vi "Channel 0 Individual Tube check (Reperpouse for Brute Force).vi"(0 "VISA Refnum in":refnum<visa-resource-name>, 1 "Test?":bool, 2 "Channel # in":i32, 3 "BoardHandle in":T1, 5 "Array":dbl[](array[numeric]), 7 "error in (no error)":errorcluster, 8 "Barcodes in":string[](array[string]), 11 "Tube #":i32) -> (12 "Next Measurment":string, 14 "Recorded Current\nfor Previous Tube":dbl format="%#_13g", 16 "Actual Voltage Level (V) 2":dbl format="%#_13g")   [LabVIEW 2020]
uses:
  <instrlib>/CAEN PSM/CAEN PSM.lvlib
panel:
  out "Failed Tubes":string[](array[string])
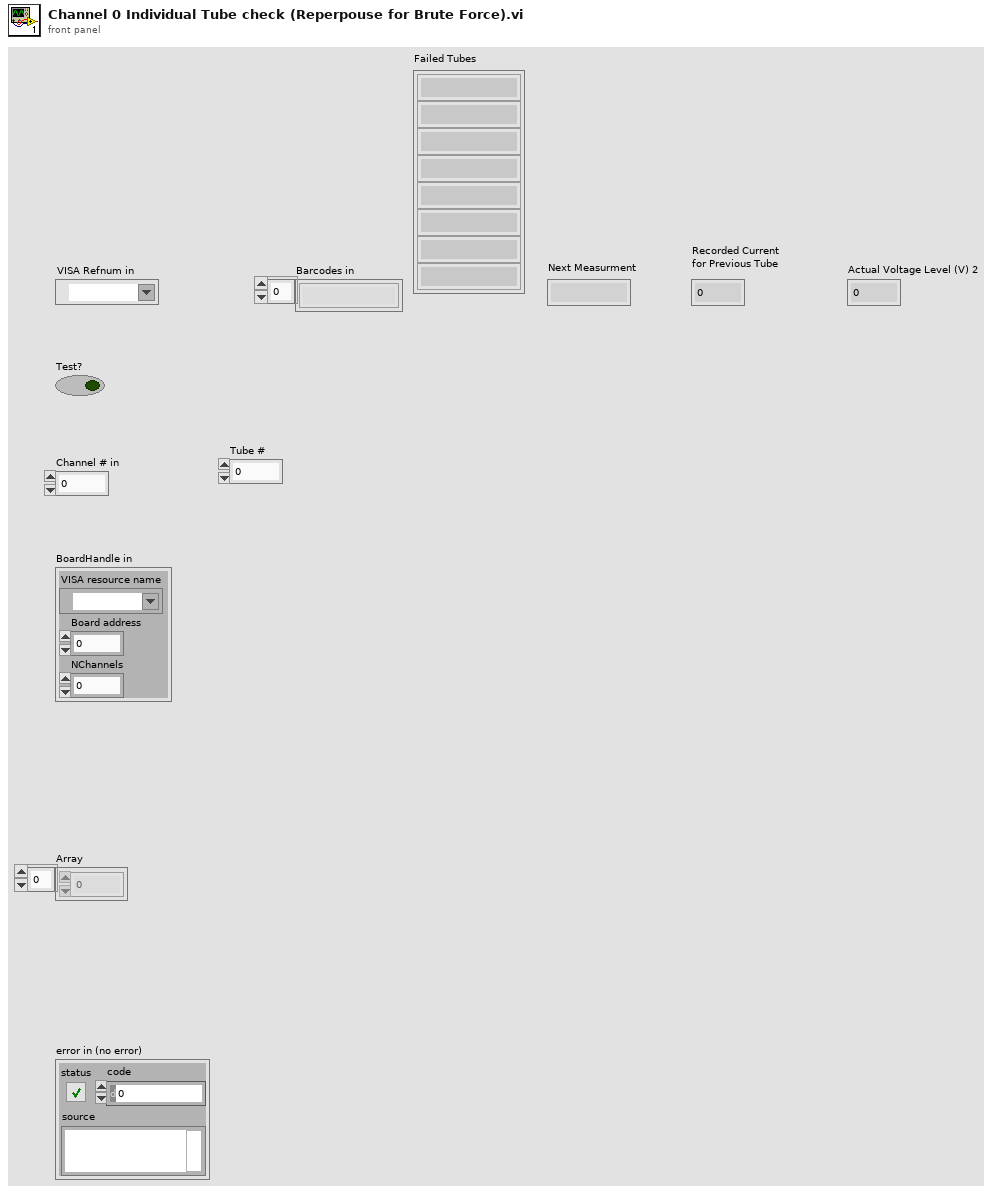
[diagram p1: front panel]
types:
  T1 = cluster{"VISA resource name":refnum<visa-resource-name>, "Board address":u8, "NChannels":u8}
  T2 = cluster{"ON":bool, "RUP":bool, "RDW":bool, "OVC":bool, "OVV":bool, "UNV":bool, "MAXV":bool, "TRIP":bool, "OVP":bool, "OVT":bool, "DIS":bool, "KILL":bool, "ILK":bool, "NOCAL":bool}[]
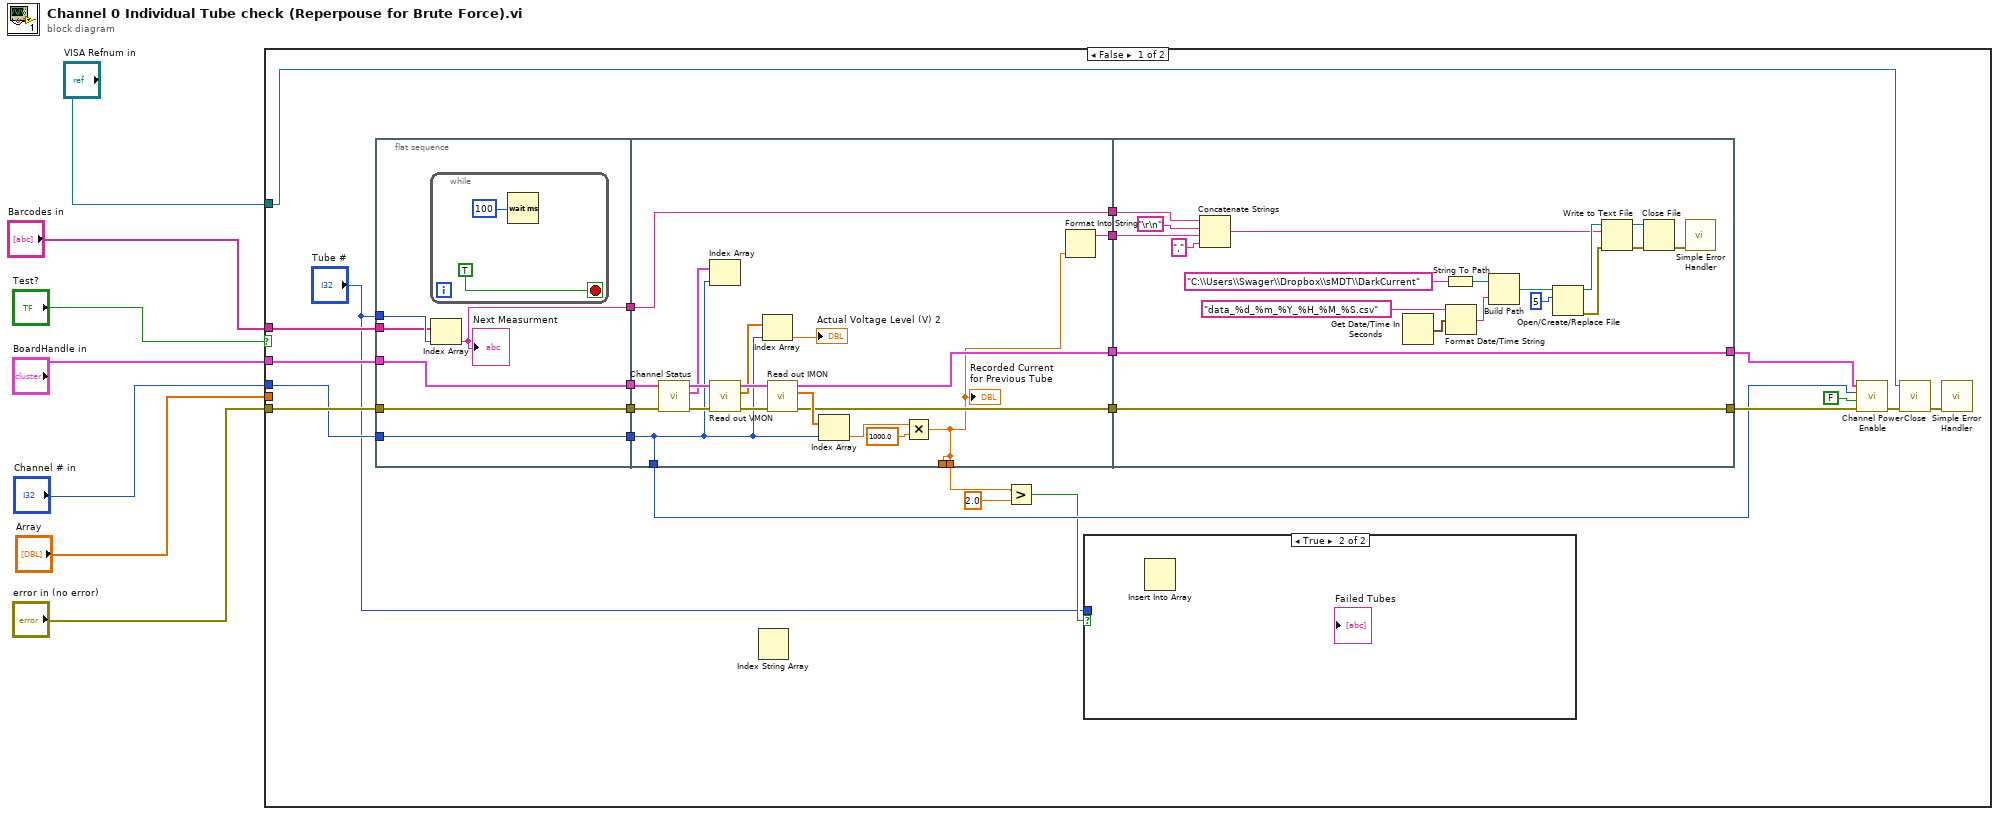
[diagram p0: block diagram]
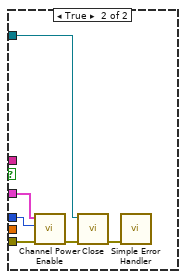
[diagram p3: hidden frame]
diagram:
  n1 = case shown="False" "Test?" {
    tunnel: "BoardHandle in" -> [w29 w78]
    tunnel: "error in (no error)" -> [w30 w77]
    tunnel: "Channel # in" -> [w28 w76]
    tunnel: "VISA Refnum in" -> [w24 w79]
    tunnel: "Array" -> [_ _]
    tunnel: "Barcodes in" -> [w20 _]
    frame False {
      n2 = flat-sequence {
        tunnel: "Tube #" -> [w36]
        tunnel: [w35] -> w19
        tunnel: w28 -> [w34]
        tunnel: [w34] -> w18
        tunnel: [w33] -> w17
        tunnel: w29 -> [w33]
        tunnel: [w32] -> w16
        tunnel: w30 -> [w32]
        tunnel: w20 -> [w31]
        tunnel: w19 -> [w46]
        tunnel: [w46] -> w15
        tunnel: w18 -> [w41]
        tunnel: w17 -> [w44]
        tunnel: w16 -> [w45]
        tunnel: [w43] -> w14
        tunnel: [w42] -> w13
        tunnel: [w41] -> w21
        tunnel: [w40] -> w12
        tunnel: [w39] -> w11
        tunnel: [w39] -> _
        tunnel: w15 -> [w61]
        tunnel: w14 -> [w59]
        tunnel: w13 -> [w58]
        tunnel: [w59] -> w23
        tunnel: [w58] -> w22
        tunnel: w12 -> [w57]
        frame #0 {
          n3 = while {
            stop <- TRUE ("Measure Next Tube") stop-if-true
            n4 = Wait (ms)(milliseconds to wait=100) -> ()  [unwired: 1 out]
          }
          n5 = Index Array(array=w31, index=w36) -> (element=w35:string)
          "Next Measurment" <- w35
        }
        frame #1 {
          n6 = call <instrlib>:"Channel Status.vi"("error in (no error)"=w45, "BoardHandle"=w44) -> ("error out"=w49:errorcluster, "Channel Status Array"=w48:T2, "BoardHandle out"=w50:T1)  [unwired: 7 in]
          n7 = Index Array(array=w48, index=w41) -> ()  [unwired: 1 out]
          n8 = call <instrlib>:"Read out VMON.vi"("error in (no error)"=w49, "BoardHandle"=w50) -> ("error out"=w53:errorcluster, "VMon values (V)"=w51:dbl[], "BoardHandle out"=w52:T1)  [unwired: 7 in]
          n9 = Index Array(array=w51, index=w41) -> (element=→"Actual Voltage Level (V) 2":dbl)
          n10 = call <instrlib>:"Read out IMON.vi"("error in (no error)"=w53, "BoardHandle"=w52) -> ("error out"=w42:errorcluster, "IMon values (uA)"=w56:dbl[], "BoardHandle out"=w43:T1)  [unwired: 6 in, 1 out]
          n11 = Index Array(array=w56, index=w41) -> (element=w54:dbl)
          n12 = Multiply(x=w54, y=1000.0) -> (x*y=w39:dbl)
          "Recorded Current\nfor Previous Tube" <- w39
          n13 = Format Into String(w39) -> (resulting string=w40:string)  [unwired: 3 in, 1 out]
        }
        frame #2 {
          n14 = Concatenate Strings(w61, "\r\n", w57, ",") -> (w63:string)
          n15 = Get Date/Time In Seconds() -> (seconds since 1Jan1904=w73:timestamp)
          n16 = String To Path(string="C:\\Users\\Swager\\Dropbox\\sMDT\\DarkCurrent") -> (path=w72:path)
          n17 = Format Date/Time String(time format string (%c)="data_%d_%m_%Y_%H_%M_%S.csv", seconds (now)=w73) -> (date/time string=w74:string)  [unwired: 1 in]
          n18 = Build Path(base path=w72, name or relative path=w74) -> (appended path=w70:path)
          n19 = Open/Create/Replace File(file path (use dialog)=w70, operation (0:open)=5) -> (refnum out=w69:refnum<file>, error out=w68:errorcluster)  [unwired: 4 in, 1 out]
          n20 = Write to Text File(file (use dialog)=w69, text=w63, error in=w68) -> (refnum out=w67:refnum<file>, error out=w66:errorcluster)  [unwired: 1 in, 1 out]
          n21 = Close File(refnum=w67, error in=w66) -> (error out=w65:errorcluster)  [unwired: 1 out]
          n22 = call <vilib>:"Simple Error Handler.vi"("error in (no error)"=w65) -> ()  [unwired: 4 in, 5 out]
        }
      }
      n23 = Index String Array() -> ()  [unwired: 3 in, 1 out]
      n24 = Greater?(x=w11, y=2.0) -> (0:w9:bool)
      n25 = case shown="True" w9 {
        tunnel: "Tube #" -> [_ _]
        frame False {
        }
        frame True {
          n26 = Insert Into Array() -> ()  [unwired: 3 in, 1 out]
        }
      }
      n27 = call <instrlib>:"Channel Power Enable.vi"("error in (no error)"=w22, "Enable (OFF)"=FALSE, "Channel (0)"=w21, "BoardHandle"=w23) -> ("error out"=w26:errorcluster)  [unwired: 6 in, 1 out]
      n28 = call <instrlib>:"Close.vi"("error in (no error)"=w26, "VISA resource name"=w24) -> ("error out"=w25:errorcluster)  [unwired: 9 in]
      n29 = call <vilib>:"Simple Error Handler.vi"("error in (no error)"=w25) -> ()  [unwired: 4 in, 5 out]
    }
    frame True {
      n30 = call <instrlib>:"Channel Power Enable.vi"("error in (no error)"=w77, "Channel (0)"=w76, "BoardHandle"=w78) -> ("error out"=w81:errorcluster)  [unwired: 7 in, 1 out]
      n31 = call <instrlib>:"Close.vi"("error in (no error)"=w81, "VISA resource name"=w79) -> ("error out"=w80:errorcluster)  [unwired: 9 in]
      n32 = call <vilib>:"Simple Error Handler.vi"("error in (no error)"=w80) -> ()  [unwired: 4 in, 5 out]
    }
  }
